vi "Motors.vi"() -> ()   [LabVIEW 2019]
uses:
  <vilib>/myRIO/Instrument Drivers/Onboard IO/PWM/typedefs/PWM Reference.ctl
  <vilib>/myRIO/Common/Instrument Driver Framework/Utilities/typedefs/myRIO Generic Hardware Reference.ctl
  <vilib>/myRIO/Common/Instrument Driver Framework/Utilities/typedefs/Hardware Version Enum.ctl
  <vilib>/myRIO/Common/Instrument Driver Framework/Utilities/typedefs/myRIO v1.0 Reference.ctl
  <vilib>/myRIO/Common/Instrument Driver Framework/Utilities/typedefs/Generic FPGA Reference.ctl
  <vilib>/myRIO/Common/Instrument Driver Framework/myRIO v1.0/PWM/typedefs/PWM Channels Enum.ctl
  <vilib>/myRIO/Instrument Drivers/Onboard IO/PWM/typedefs/PWM Configuration.ctl
  <vilib>/userdefined/High Color/nirio_resource_hc.ctl
  <vilib>/myRIO/Common/Instrument Driver Framework/myRIO v1.0/PWM/vis/myRIO v1.1 Open PWM.vi
  <vilib>/myRIO/Common/Instrument Driver Framework/Utilities/vis/Validate Channels.vi
  <vilib>/myRIO/Common/Instrument Driver Framework/myRIO v1.0/PWM/vis/myRIO v1.0 Reserve PWM.vi
  <vilib>/myRIO/Common/Instrument Driver Framework/myRIO v1.0/PWM/vis/myRIO v1.0 Close PWM.vi
  <vilib>/myRIO/Common/Instrument Driver Framework/myRIO v1.0/PWM/vis/myRIO v1.0 Build MUX Configuration PWM.vi
  <vilib>/myRIO/Common/Instrument Driver Framework/myRIO v1.0/Resource Manager/vis/myRIO v1.0 Reserve Channel List.vi
  <vilib>/myRIO/Common/Instrument Driver Framework/myRIO v1.0/PWM/vis/myRIO v1.0 Unreserve PWM.vi
  <vilib>/myRIO/Common/Instrument Driver Framework/myRIO v1.0/Resource Manager/vis/myRIO v1.0 Create Configuration List.vi
  <vilib>/myRIO/Common/Instrument Driver Framework/myRIO v1.0/Resource Manager/vis/myRIO v1.0 Reserve Channel.vi
  <vilib>/myRIO/Common/Instrument Driver Framework/myRIO v1.0/Resource Manager/vis/myRIO v1.0 Unreserve Channel.vi
  <vilib>/myRIO/Common/Instrument Driver Framework/myRIO v1.0/Resource Manager/vis/myRIO v1.0 Unreserve Channel List.vi
  <vilib>/myRIO/Common/Instrument Driver Framework/myRIO v1.0/Resource Manager/vis/myRIO v1.0 Build Mutex Name.vi
  <vilib>/Utility/VariantDataType/GetNumericInfo.vi
  <vilib>/Utility/error.llb/Error Cluster From Error Code.vi
  <vilib>/myRIO/Common/Instrument Driver Framework/myRIO v1.0/myRIO v1.1 Open.vi
  <vilib>/myRIO/Common/Instrument Driver Framework/Utilities/vis/IO Manager.vi
  <vilib>/myRIO/Common/Instrument Driver Framework/Utilities/vis/Configuration Manager.vi
  <vilib>/myRIO/Common/Instrument Driver Framework/myRIO v1.0/Resource Manager/vis/myRIO v1.0 Configure IO.vi
  <vilib>/myRIO/Common/Instrument Driver Framework/myRIO v1.0/myRIO v1.0 Close.vi
  <vilib>/myRIO/Common/Instrument Driver Framework/myRIO v1.0/PWM/vis/myRIO v1.0 Write PWM.vi
  <vilib>/myRIO/Common/Instrument Driver Framework/myRIO v1.0/PWM/vis/myRIO v1.0 Shutdown PWM.vi
  <vilib>/myRIO/Instrument Drivers/Onboard IO/PWM/vis/myRIO PWM Open.xnode
  <vilib>/myRIO/Instrument Drivers/Onboard IO/PWM/PWM.lvlib
panel:
  in  "STOP RIGHT MOTOR":bool
  in  "RIGHT MOTOR DUTY CYCLE":dbl(slide)=50.00000000000001 scale=0.0..100.0
  in  "STOP LEFT MOTOR":bool
  in  "LEFT MOTOR DUTY CYCLE":dbl(slide)=50.00000000000001 scale=0.0..100.0
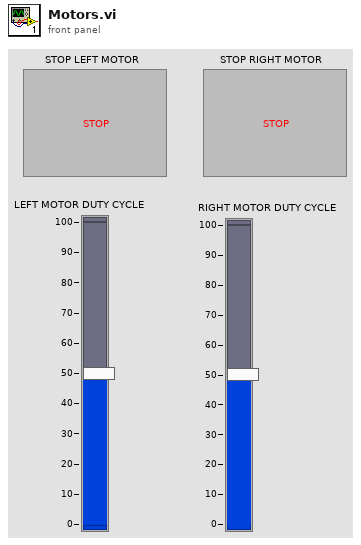
[diagram p1: front panel]
types:
  T1 = typedef "PWM.lvlib/PWM Reference.ctl" = cluster{"myRIO Reference":T2, "PWM Channels Enum":T6, "PWM Configuration":T7}
  T2 = typedef "myRIO Generic Hardware Reference.ctl" = cluster{"myRIO Model":T3, "myRIO Hardware Reference":T4}
  T3 = typedef "Hardware Version Enum.ctl" = enum16{"Unknown", "myRIO-1900", "myRIO-1950", "roboRIO", "NI ELVIS RIO CM", "ELVIS III"}
  T4 = typedef "myRIO v1.0 Reference.ctl" = cluster{"Generic FPGA Reference":T5, "Allow multiple opens":bool}
  T5 = typedef "Generic FPGA Reference.ctl" = refnum<k20>
  T6 = typedef "PWM Channels Enum.ctl" = enum16{"Not Connected", "C/PWM0", "C/PWM1", "A/PWM0", "A/PWM1", "A/PWM2", "A/PWM3", "A/PWM4", "A/PWM5", "A/PWM6", "A/PWM7", "A/PWM8", "A/PWM9", "A/PWM10", "A/PWM11", "A/PWM12", "A/PWM13", "A/PWM14", "A/PWM15", "A/PWM16", "A/PWM17", "A/PWM18", "A/PWM19", "B/PWM0", "B/PWM1", "B/PWM2", "B/PWM3", "B/PWM4", "B/PWM5", "B/PWM6", "B/PWM7", "B/PWM8", "B/PWM9", "B/PWM10", "B/PWM11", "B/PWM12", "B/PWM13", "B/PWM14", "B/PWM15", "B/PWM16", "B/PWM17", "B/PWM18", "B/PWM19", "PWM/PWM0", "PWM/PWM1", "PWM/PWM2", "PWM/PWM3", "PWM/PWM4", "PWM/PWM5", "PWM/PWM6", "PWM/PWM7", "PWM/PWM8", "PWM/PWM9"}
  T7 = typedef "PWM.lvlib/PWM Configuration.ctl" = cluster{"Frequency":dbl, "Duty Cycle":dbl}
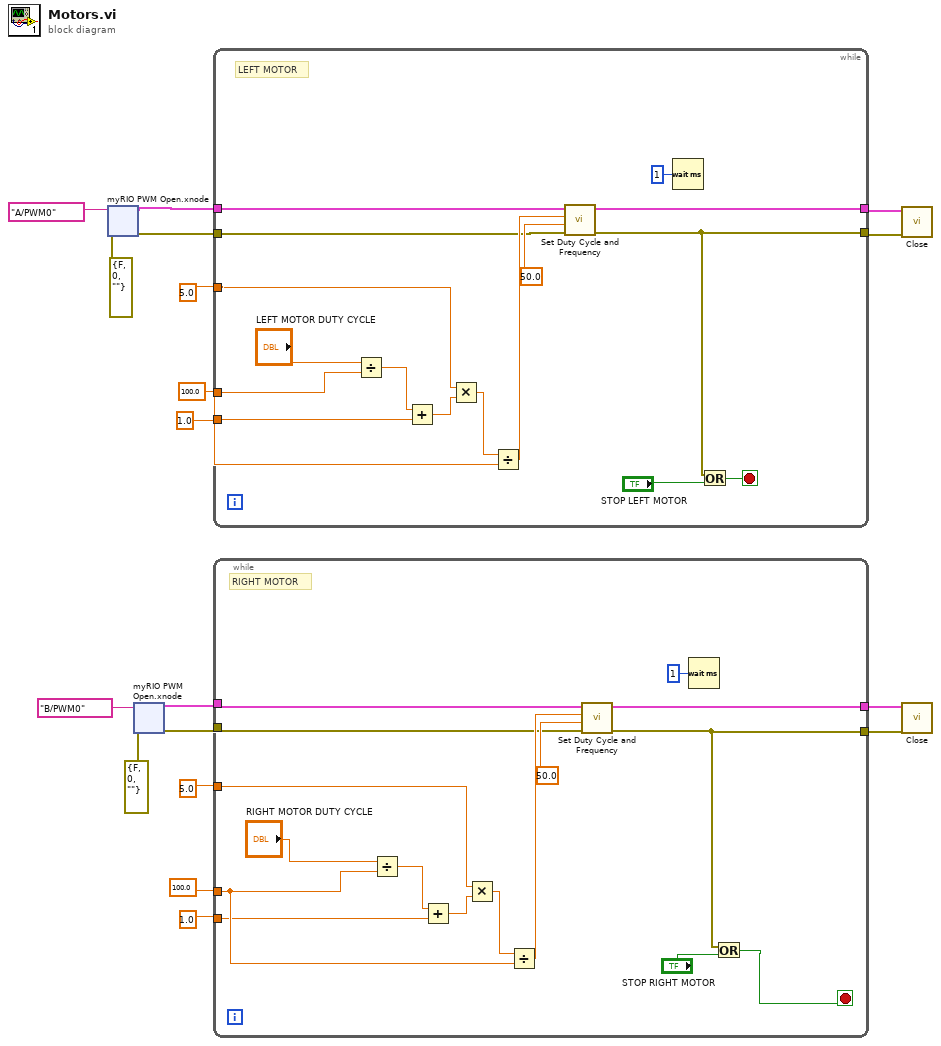
[diagram p0: block diagram]
diagram:
  n1 = xnode "myRIO PWM Open.xnode"("error in (no error)"=errorcluster {"status"=FALSE, "code"=0, "source"=""}, "Channel Name"=tag "A/PWM0") -> ("error out"=w15:errorcluster, "PWM Ref Out"=w2:T1)  [unwired: 1 in]
  n2 = xnode "myRIO PWM Open.xnode"("error in (no error)"=errorcluster {"status"=FALSE, "code"=0, "source"=""}, "Channel Name"=tag "B/PWM0") -> ("error out"=w1:errorcluster, "PWM Ref Out"=w4:T1)  [unwired: 1 in]
  n3 = while {
    tunnel: w2 -> [w28]
    tunnel: [w27] -> w14
    tunnel: [w20] -> w3
    tunnel: w15 -> [w26]
    tunnel: 5.0 ("Numeric 2") -> [w25]
    tunnel: 100.0 ("Numeric") -> [w24]
    tunnel: 1.0 ("Numeric 3") -> [w23]
    stop <- w21 stop-if-true
    # "LEFT MOTOR"
    n4 = Divide(x="LEFT MOTOR DUTY CYCLE", y=w24) -> (x/y=w29:dbl)
    n5 = Add(x=w29, y=w23) -> (x+y=w30:dbl)
    n6 = Multiply(x=w25, y=w30) -> (x*y=w31:dbl)
    n7 = Divide(x=w31, y=w24) -> (x/y=w33:dbl)
    n8 = call <vilib>:"Set Duty Cycle and Frequency.vi"("error in (no error)"=w26, "Frequency [Hz]"=50.0, "Duty Cycle"=w33, "PWM Ref In"=w28) -> ("error out"=w20:errorcluster, "PWM Ref Out"=w27:T1)  [unwired: 5 in]
    n9 = Wait (ms)(milliseconds to wait=u32 1) -> ()  [unwired: 1 out]
    n10 = Or(x=w20, y="STOP LEFT MOTOR") -> (x .or. y?=w21:bool)
  }
  n11 = while {
    tunnel: w4 -> [w44]
    tunnel: [w43] -> w9
    tunnel: [w35] -> w8
    tunnel: w1 -> [w42]
    tunnel: 5.0 ("Numeric 2") -> [w41]
    tunnel: 100.0 ("Numeric") -> [w40]
    tunnel: 1.0 ("Numeric 3") -> [w39]
    stop <- w36 stop-if-true
    # "RIGHT MOTOR"
    n12 = Divide(x="RIGHT MOTOR DUTY CYCLE", y=w40) -> (x/y=w45:dbl)
    n13 = Add(x=w45, y=w39) -> (x+y=w46:dbl)
    n14 = Multiply(x=w41, y=w46) -> (x*y=w47:dbl)
    n15 = Divide(x=w47, y=w40) -> (x/y=w49:dbl)
    n16 = call <vilib>:"Set Duty Cycle and Frequency.vi"("error in (no error)"=w42, "Frequency [Hz]"=50.0, "Duty Cycle"=w49, "PWM Ref In"=w44) -> ("error out"=w35:errorcluster, "PWM Ref Out"=w43:T1)  [unwired: 5 in]
    n17 = Wait (ms)(milliseconds to wait=u32 1) -> ()  [unwired: 1 out]
    n18 = Or(x=w35, y="STOP RIGHT MOTOR") -> (x .or. y?=w36:bool)
  }
  n19 = call <vilib>:"Close.vi"("error in (no error)"=w3, "PWM Ref In"=w14) -> ()  [unwired: 9 in, 1 out]
  n20 = call <vilib>:"Close.vi"("error in (no error)"=w8, "PWM Ref In"=w9) -> ()  [unwired: 9 in, 1 out]
